vi "QI radial profile calculate_C.vi"(7 "r":dbl, 8 "rad":dbl[](array[numeric]), 9 "Yr":dbl, 10 "Xr":dbl, 11 "ROI array":sgl[][](array[numeric])) -> (0 "mean4":dbl, 1 "mean3":dbl, 2 "mean2":dbl, 3 "mean1":dbl)   [LabVIEW 2017]
panel:
  in  "num":i32
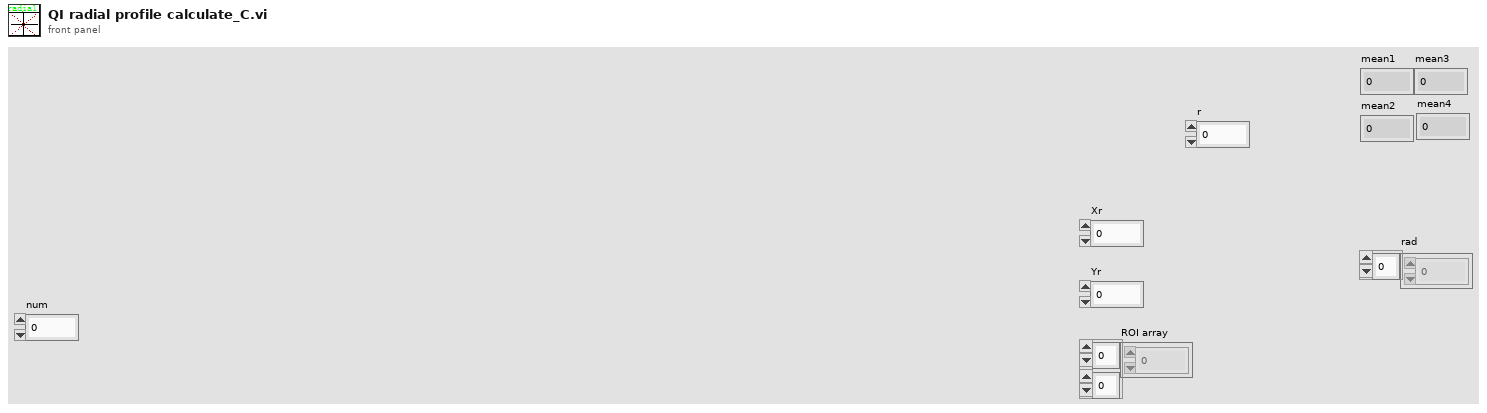
[diagram p1: front panel]
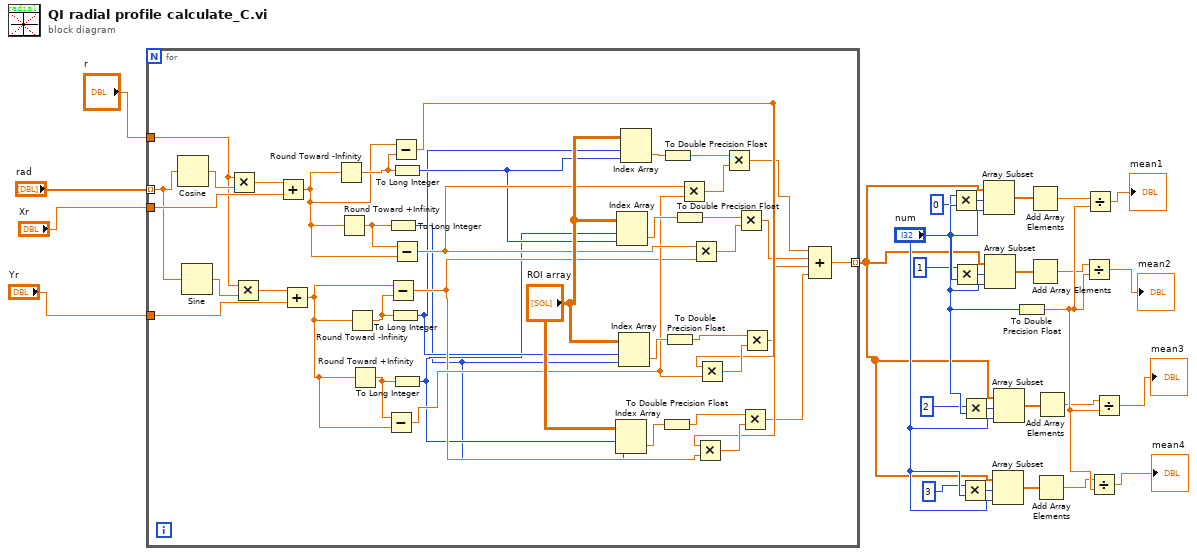
[diagram p0: block diagram]
diagram:
  n1 = for {
    tunnel: "Xr" -> [w67]
    tunnel: "r" -> [w60]
    tunnel: "rad" -> [w62] mode=indexing
    tunnel: "Yr" -> [w61]
    tunnel: [w32] -> w9 mode=indexing
    n2 = Cosine(x=w62) -> (cos(x)=w65:dbl)
    n3 = Sine(x=w62) -> (sin(x)=w64:dbl)
    n4 = Multiply(x=w60, y=w65) -> (x*y=w66:dbl)
    n5 = Multiply(x=w60, y=w64) -> (x*y=w63:dbl)
    n6 = Add(x=w66, y=w67) -> (x+y=w55:dbl)
    n7 = Add(x=w63, y=w61) -> (x+y=w53:dbl)
    n8 = Round Toward -Infinity(1:w55) -> (0:w57:dbl)
    n9 = Round Toward +Infinity(x=w55) -> (ceil(x): smallest int >= x=w56:dbl)
    n10 = Round Toward -Infinity(1:w53) -> (0:w54:dbl)
    n11 = Round Toward +Infinity(x=w53) -> (ceil(x): smallest int >= x=w52:dbl)
    n12 = Subtract(x=w52, y=w53) -> (x-y=w41:dbl)
    n13 = To Long Integer(number=w56) -> (32bit integer=w28:i32)
    n14 = Subtract(x=w53, y=w54) -> (x-y=w37:dbl)
    n15 = To Long Integer(number=w54) -> (32bit integer=w30:i32)
    n16 = Subtract(x=w55, y=w57) -> (x-y=w38:dbl)
    n17 = To Long Integer(number=w57) -> (32bit integer=w31:i32)
    n18 = Subtract(x=w56, y=w55) -> (x-y=w44:dbl)
    n19 = To Long Integer(number=w52) -> (32bit integer=w29:i32)
    n20 = Index Array(array="ROI array", index (row)=w29, index (col)=w28) -> (element=w40:sgl)
    n21 = Index Array(array="ROI array", index (row)=w29, index (col)=w31) -> (element=w46:sgl)
    n22 = Index Array(array="ROI array", index (row)=w30, index (col)=w28) -> (element=w43:sgl)
    n23 = Index Array(array="ROI array", index (row)=w30, index (col)=w31) -> (element=w59:sgl)
    n24 = To Double Precision Float(number=w40) -> (double precision float=w39:dbl)
    n25 = To Double Precision Float(number=w59) -> (double precision float=w51:dbl)
    n26 = To Double Precision Float(number=w43) -> (double precision float=w42:dbl)
    n27 = To Double Precision Float(number=w46) -> (double precision float=w45:dbl)
    n28 = Multiply(x=w44, y=w41) -> (x*y=w50:dbl)
    n29 = Multiply(x=w44, y=w37) -> (x*y=w49:dbl)
    n30 = Multiply(x=w38, y=w37) -> (x*y=w47:dbl)
    n31 = Multiply(x=w38, y=w41) -> (x*y=w48:dbl)
    n32 = Multiply(x=w51, y=w50) -> (x*y=w36:dbl)
    n33 = Multiply(x=w45, y=w49) -> (x*y=w35:dbl)
    n34 = Multiply(x=w39, y=w47) -> (x*y=w33:dbl)
    n35 = Multiply(x=w42, y=w48) -> (x*y=w34:dbl)
    n36 = Compound Arithmetic op=ADD(w36, w35, w34, w33) -> (w32:dbl)
  }
  n37 = Multiply(x=0 ("索引"), y="num") -> (x*y=w10:i32)
  n38 = Multiply(x=1 ("索引"), y="num") -> (x*y=w11:i32)
  n39 = Multiply(x=3 ("索引"), y="num") -> (x*y=w13:i32)
  n40 = Multiply(x=2 ("索引"), y="num") -> (x*y=w12:i32)
  n41 = Array Subset(array=w9, index=w10, length="num") -> (w14:dbl[])
  n42 = Array Subset(array=w9, index=w11, length="num") -> (w15:dbl[])
  n43 = Array Subset(array=w9, index=w13, length="num") -> (w17:dbl[])
  n44 = Array Subset(array=w9, index=w12, length="num") -> (w16:dbl[])
  n45 = To Double Precision Float(number="num") -> (double precision float=w23:dbl)
  n46 = Add Array Elements(numeric array=w14) -> (sum=w20:dbl)
  n47 = Add Array Elements(numeric array=w15) -> (sum=w18:dbl)
  n48 = Add Array Elements(numeric array=w17) -> (sum=w21:dbl)
  n49 = Add Array Elements(numeric array=w16) -> (sum=w22:dbl)
  n50 = Divide(x=w18, y=w23) -> (x/y=→"mean2":dbl)
  n51 = Divide(x=w20, y=w23) -> (x/y=→"mean1":dbl)
  n52 = Divide(x=w21, y=w23) -> (x/y=→"mean4":dbl)
  n53 = Divide(x=w22, y=w23) -> (x/y=→"mean3":dbl)
